vi "Utility Generate Instrument Error.vi"(0 "VISA resource name":refnum<visa-resource-name>, 5 "Status (F: Off)":bool, 9 "Code (0)":i32 format="%.0x", 11 "error in (no error)":errorcluster {"code" format="%.0x"}) -> (4 "VISA resource name out":refnum<visa-resource-name>, 15 "error out":errorcluster {"code" format="%.0x"})   [LabVIEW 2010, in "Eurotherm 32xx Series.lvlib"]
doc: "This VI generates the error cluster with Error Code as code and chain of VI as source. The source does not include the name of this VI."
uses:
  <instrlib>/Eurotherm 32xx Series/Eurotherm 32xx Series.lvlib
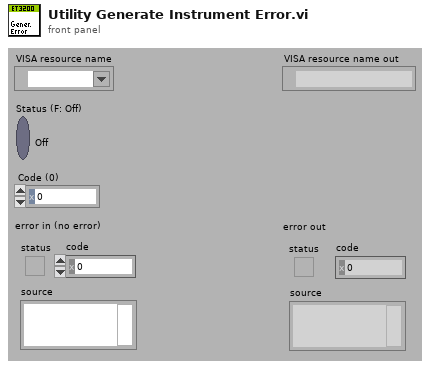
[diagram p1: front panel]
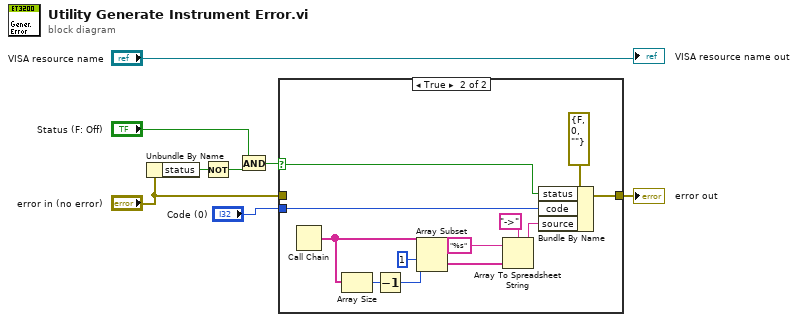
[diagram p0: block diagram]
diagram:
  n1 = Unbundle By Name("error in (no error)") -> ("status"=w8:bool)
  n2 = Not(x=w8) -> (.not. x?=w6:bool)
  n3 = And(x="Status (F: Off)", y=w6) -> (x .and. y?=w4:bool)
  n4 = case shown="True" w4 {
    selector: w4 -> [_ w12]
    tunnel: [w9 w13] -> w7
    tunnel: "error in (no error)" -> [w9 _]
    tunnel: "Code (0)" -> [_ w10]
    frame False {
    }
    frame True {
      n5 = Call Chain() -> (call chain=w20:string[])
      n6 = Array Size(array=w20) -> (size(s)=w19:i32)
      n7 = Decrement(x=w19) -> (x-1=w18:i32)
      n8 = Array Subset(array=w20, index=1 ("Array Index"), length=w18) -> (w11:string[])
      n9 = Array To Spreadsheet String(delimiter (Tab)="->", array=w11, 3:"%s" ("format string")) -> (spreadsheet string=w14:string)
      n10 = Bundle By Name(cluster=errorcluster {"status"=FALSE, "code"=0, "source"=""} ("Error Out"), "status"=w12, "code"=w10, "source"=w14) -> (w13:errorcluster)
    }
  }
  "error out" <- w7
  "VISA resource name out" <- "VISA resource name"
